vi "07.1 Loop basics.vi"() -> ()   [LabVIEW 2019]
panel:
  in  "stop 3":bool
  out "Waveform Chart":dbl(graph)
  in  "stop 2":bool
  out "for loop iteration":i32
  out "Random Number":dbl
  out "final iteration":i32
  in  "stop":bool
  out "while loop iterations":i32
  out "minutes":dbl
  out "seconds":dbl
  out "hours":dbl
  in  "total time (s)":dbl
  # "While loop"
  # "For loop"
  # "Timing loops"
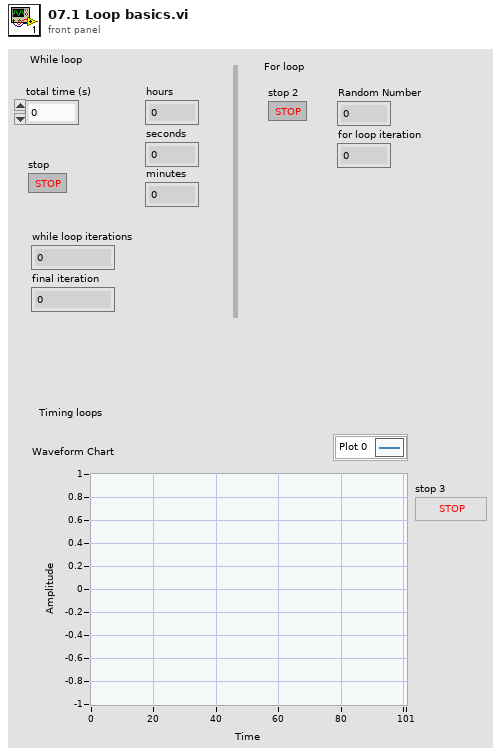
[diagram p1: front panel]
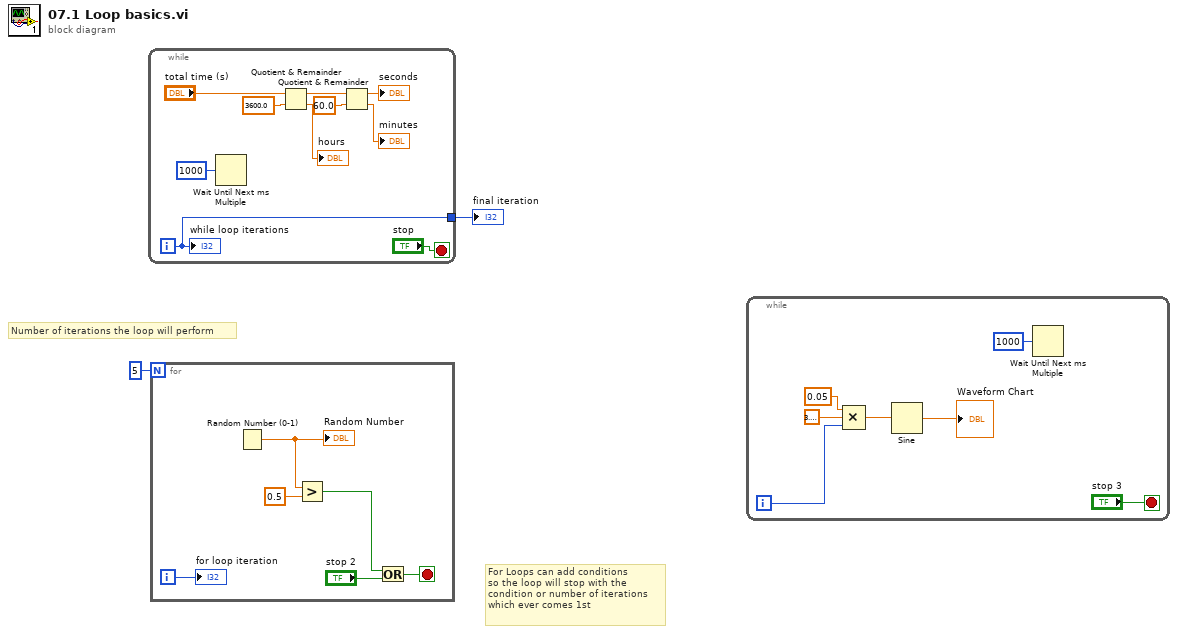
[diagram p0: block diagram]
diagram:
  # "For Loops can add conditions\nso the loop will stop with the \ncondition or number of iterations\nwhich ever comes 1st"
  # "Number of iterations the loop will perform"
  n1 = while {
    tunnel: [w4] -> w2
    i -> [w4]
    stop <- "stop" stop-if-true
    n2 = Wait Until Next ms Multiple(millisecond multiple=u32 1000) -> ()  [unwired: 1 out]
    n3 = Quotient & Remainder(x="total time (s)", y=3600.0) -> (x-y*floor(x/y)=w8:dbl, floor(x/y)=→"hours":dbl)
    n4 = Quotient & Remainder(x=w8, y=60.0) -> (x-y*floor(x/y)=→"seconds":dbl, floor(x/y)=→"minutes":dbl)
    "while loop iterations" <- w4
  }
  "final iteration" <- w2
  n5 = for {
    N: 5 -> [_]
    i -> [w18]
    stop <- w14 stop-if-true
    n6 = Random Number (0-1)() -> (number: 0 to 1=w17:dbl)
    "Random Number" <- w17
    n7 = Greater?(x=w17, y=0.5) -> (0:w13:bool)
    n8 = Or(x=w13, y="stop 2") -> (x .or. y?=w14:bool)
    "for loop iteration" <- w18
  }
  n9 = while {
    i -> [w22]
    stop <- "stop 3" stop-if-true
    n10 = Compound Arithmetic op=MULTIPLY(0.05 ("value"), 3.141592653589793, w22) -> (w20:dbl)
    n11 = Sine(x=w20) -> (sin(x)=→"Waveform Chart":dbl)
    n12 = Wait Until Next ms Multiple(millisecond multiple=u32 1000) -> ()  [unwired: 1 out]
  }
